vi "Evaluate Gradient.vi"(2 "Point (x_1, ..., x_n)":dbl[](array[numeric]), 4 "Function Reference":refnum<vi>) -> (0 "Gradient":dbl[](array[numeric]))   [LabVIEW 2020, in "Automatic Differentiation.lvlib"]
uses:
  Automatic Differentiation.lvlib
  classes/Dual/Dual.lvclass
  classes/Dual/Dual.lvclass/Dual.ctl
  3428a883-4abf-4854-9978-3fd53a24097c.vi
  3428a883-4abf-4854-9978-3fd53a24097c.vi/5957e011-cf56-4527-b6ed-13c3a4ca997b.vi
  classes/Dual/Write a.vi
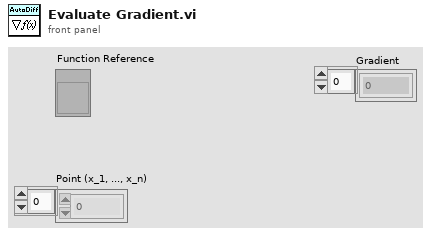
[diagram p1: front panel]
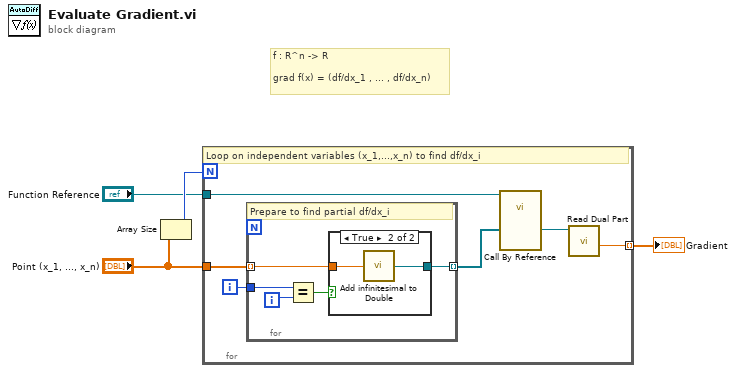
[diagram p0: block diagram]
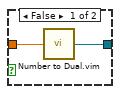
[diagram p2: hidden frame]
diagram:
  # "f : R^n -> R\n\ngrad f(x) = (df/dx_1 , ... , df/dx_n)"
  n1 = Array Size(array="Point (x_1, ..., x_n)") -> (size(s)=w4:i32)
  n2 = for {
    N: w4 -> [_]
    tunnel: "Function Reference" -> [w10]
    tunnel: "Point (x_1, ..., x_n)" -> [w8]
    tunnel: [w5] -> w3 mode=indexing
    i -> [w7]
    # "Loop on independent variables (x_1,...,x_n) to find df/dx_i"
    n3 = for {
      tunnel: w7 -> [w15]
      tunnel: w8 -> [w13] mode=indexing
      tunnel: [w11] -> w9 mode=indexing
      i -> [w14]
      # "Prepare to find partial df/dx_i"
      n4 = Equal?(x=w15, y=w14) -> (x = y?=w12:bool)
      n5 = case shown="True" w12 {
        tunnel: w13 -> [w17 w19]
        tunnel: [w16 w18] -> w11
        frame False {
          n6 = call "Number to Dual.vim"("Number"=w17) -> ("Dual"=w16:refnum<class "Dual.lvclass">)
        }
        frame True {
          n7 = call "Add infinitesimal to Double.vi"("DBL (x)"=w19) -> ("Dual (x+e)"=w18:refnum<class "Dual.lvclass">)
        }
      }
    }
    n8 = call-by-ref "?"(reference=w10, "(x_1, ..., x_n)"=w9) -> ("f(x_1, ..., x_n)"=w6:refnum<class "Dual.lvclass">)  [unwired: 1 in, 2 out]
    n9 = call "Read Dual Part.vi"("Dual in"=w6) -> ("Dual Part"=w5:dbl)  [unwired: 9 in, 1 out]
  }
  "Gradient" <- w3
